vi "Read Request.vi"(11 "Processing In":refnum<class "Processing.lvclass">) -> (0 "error out":errorcluster, 3 "HTTP Server.lvlib:Processing":refnum<class "Processing.lvclass">)   [LabVIEW 2020, in "HTTP Server.lvlib" / "Server.lvclass"]
uses:
  Server.lvclass
  Server.lvclass/Server.ctl
  lv-http-util/HTTP Utils/Request/Request.lvclass
  RequestTraceLog/RequestTraceLog.lvclass
  Processing/Processing.lvclass
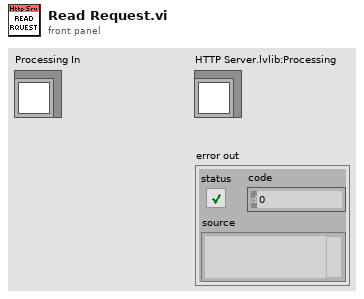
[diagram p1: front panel]
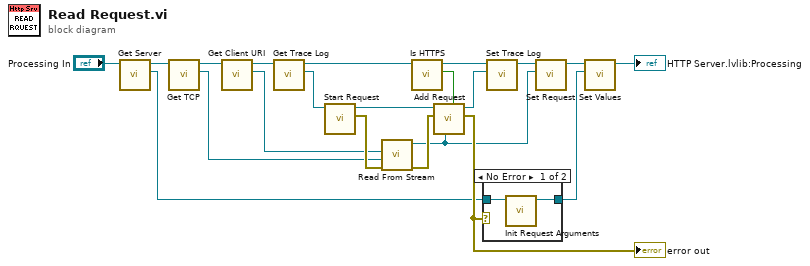
[diagram p0: block diagram]
diagram:
  n1 = call "Get Server.vi"("Processing in"="Processing In") -> ("Server"=w17:refnum<class "Server.lvclass">, "Processing out"=w8:refnum<class "Processing.lvclass">)  [unwired: 9 in]
  n2 = call "Get TCP.vi"("Processing in"=w8) -> ("TCP"=w3:refnum<k5>, "Processing out"=w9:refnum<class "Processing.lvclass">)  [unwired: 9 in]
  n3 = call "Get Client URI.vi"("Processing in"=w9) -> ("Client URI"=w1:refnum<class "URI.lvclass">, "Processing out"=w2:refnum<class "Processing.lvclass">)  [unwired: 9 in]
  n4 = call "Get Trace Log.vi"("Processing in"=w2) -> ("Trace Log"=w16:refnum<class "RequestTraceLog.lvclass">, "Processing out"=w6:refnum<class "Processing.lvclass">)  [unwired: 9 in]
  n5 = call "Start Request.vi"("RequestTraceLog in"=w16) -> ("error out"=w20:errorcluster, "RequestTraceLog out"=w18:refnum<class "RequestTraceLog.lvclass">)  [unwired: 9 in]
  n6 = call "Read From Stream.vi"("error in (no error)"=w20, "TCP in"=w3, "Client URI"=w1) -> ("error out"=w19:errorcluster, "Request out"=w13:refnum<class "Request.lvclass">)  [unwired: 6 in, 1 out]
  n7 = call "Is HTTPS.vi"("Processing in"=w6) -> ("HTTPS?"=w4:bool, "Processing out"=w5:refnum<class "Processing.lvclass">)  [unwired: 8 in, 1 out]
  n8 = call "Add Request.vi"("HTTPS?"=w4, "Request"=w13, "error in (no error)"=w19, "RequestTraceLog in"=w18) -> ("error out"=w21:errorcluster, "RequestTraceLog out"=w15:refnum<class "RequestTraceLog.lvclass">)  [unwired: 6 in]
  "error out" <- w21
  n9 = case shown="No Error" w21 {
    tunnel: [w22 _] -> w11
    tunnel: w17 -> [w23 _]
    frame No Error {
      n10 = call "Init Request Arguments.vi"("Server in"=w23) -> ("Arguments"=w22:refnum<class "Values.lvclass">)  [unwired: 9 in, 1 out]
    }
    frame Error {
    }
  }
  n11 = call "Set Trace Log.vi"("Trace Log"=w15, "Processing in"=w5) -> ("Processing out"=w14:refnum<class "Processing.lvclass">)  [unwired: 9 in]
  n12 = call "Set Request.vi"("Request"=w13, "Processing in"=w14) -> ("Processing out"=w12:refnum<class "Processing.lvclass">)  [unwired: 9 in]
  n13 = call "Set Values.vi"("Values"=w11, "Processing in"=w12) -> ("Processing out"=→"HTTP Server.lvlib:Processing":refnum<class "Processing.lvclass">)  [unwired: 9 in]
